vi "Search.vi"(8 "error in (no error)":errorcluster, 9 "SearchMethod":T1, 11 "MultiTree in":refnum<class "MultiTree.lvclass">) -> (0 "error out":errorcluster, 1 "found":bool, 2 "Node":refnum<data-value>, 3 "MultiTree out":refnum<class "MultiTree.lvclass">)   [LabVIEW 2014, in "MultiTree.lvlib" / "MultiTree.lvclass"]
uses:
  <userlib>/AdvancedDataStructures/ClassBased/MultiTree/MultiTree.lvclass
  <userlib>/AdvancedDataStructures/ClassBased/MultiTreeNode/MultiTreeNode.lvclass
  <userlib>/AdvancedDataStructures/ClassBased/MultiTree/SearchMethod.ctl
  <userlib>/AdvancedDataStructures/ClassBased/MultiTree/MultiTree.lvclass/MultiTree.ctl
  <userlib>/AdvancedDataStructures/ClassBased/MultiTreeNode/MultiTreeNode.lvclass/MultiTreeNode.ctl
  <userlib>/AdvancedDataStructures/ClassBased/LinkedList/LinkedList.lvclass
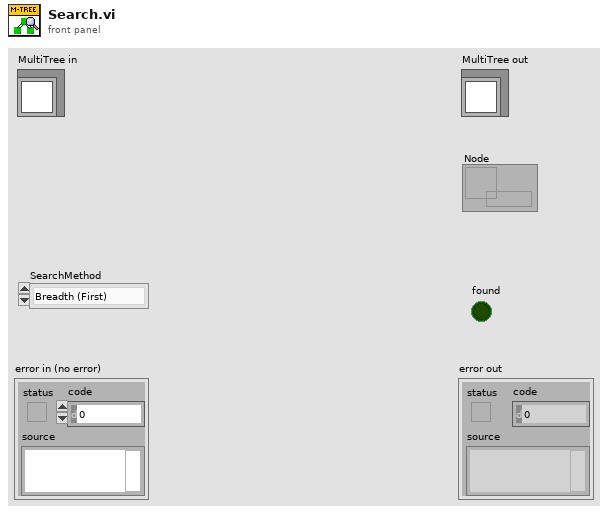
[diagram p1: front panel]
types:
  T1 = typedef "MultiTree.lvlib/MultiTree.lvclass/SearchMethod.ctl" = enum16{"Breadth (First)", "Depth (First)", "Best First", "Breadth (Exhaustive)", "Depth (Exhaustive)"}
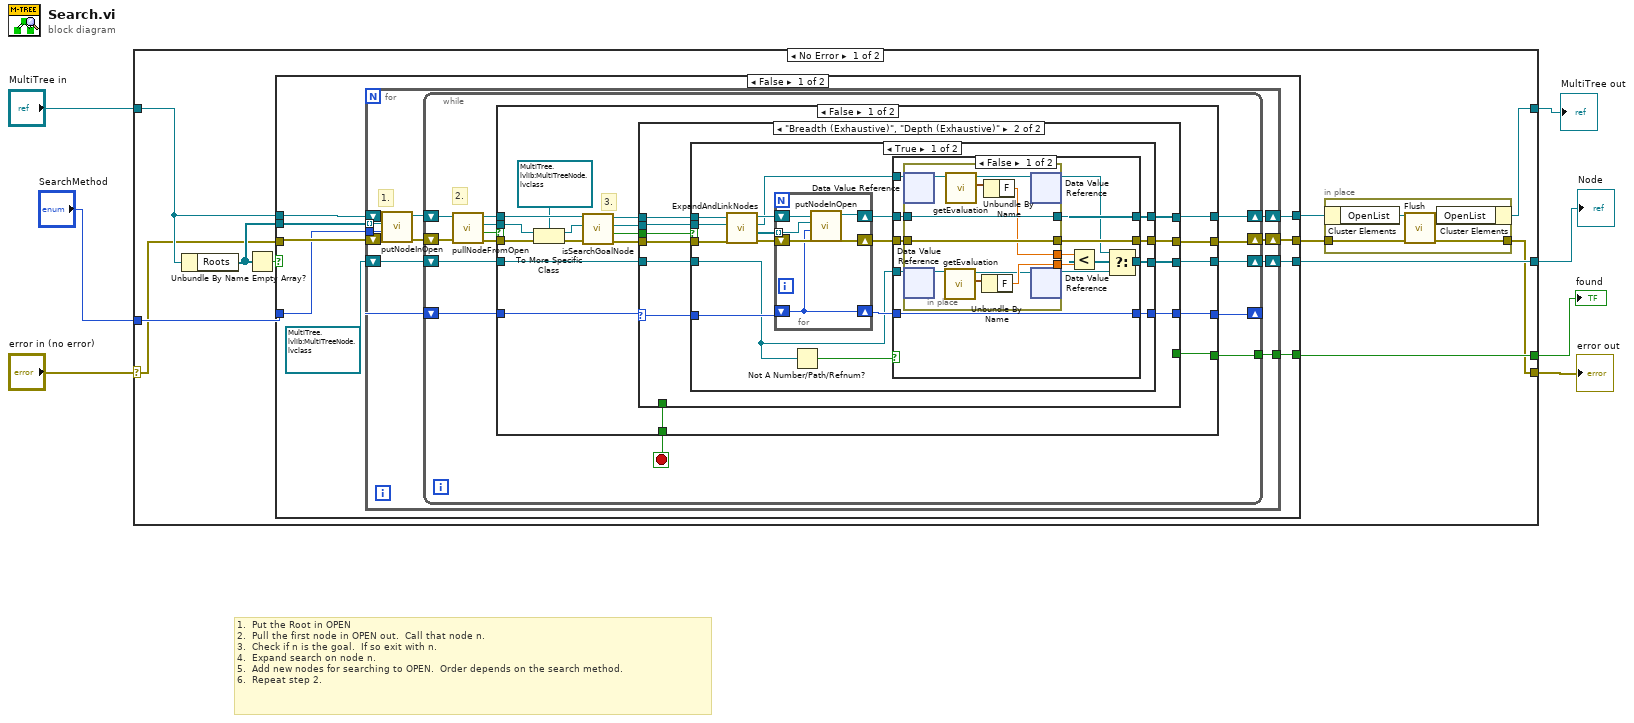
[diagram p0: block diagram]
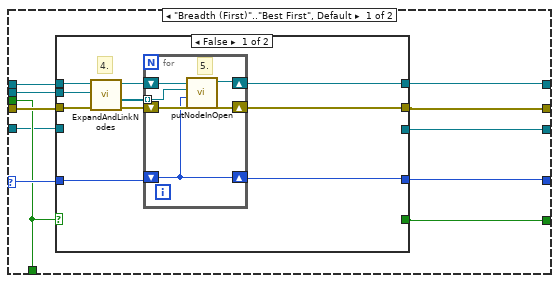
[diagram p2: hidden frame]
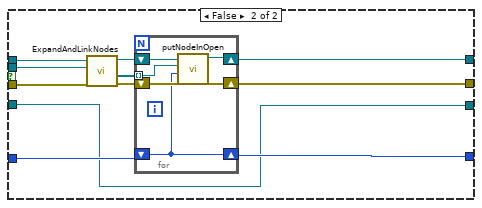
[diagram p5: hidden frame]
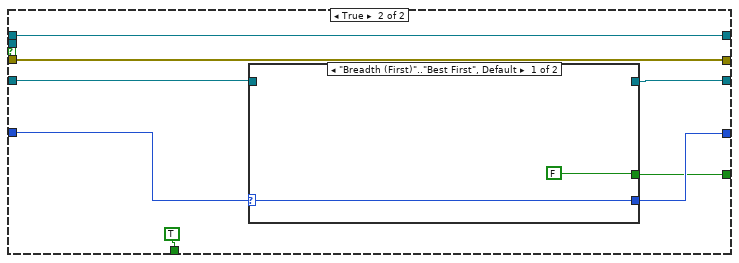
[diagram p6: hidden frame]
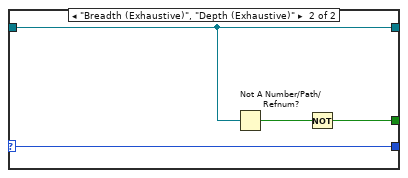
[diagram p7: hidden frame]
diagram:
  # "1.  Put the Root in OPEN\n2.  Pull the first node in OPEN out.  Call that node n.\n3.  Check if n is the goal.  If so exit with n.\n4.  Expand search on node n.\n5.  Add new nodes for searching to OPEN.  Order depends on the search method.\n6.  Repeat step 2."
  n1 = case shown="No Error" "error in (no error)" {
    selector: "error in (no error)" -> [w12 w201]
    tunnel: [w8 w201] -> w6
    tunnel: [w11 w200] -> w4
    tunnel: "MultiTree in" -> [w14 w200]
    tunnel: "SearchMethod" -> [w13 _]
    tunnel: [w10 _] -> w2
    tunnel: [w9 _] -> w1
    frame No Error {
      n2 = Unbundle By Name(w14) -> ("Roots"=w17:refnum<data-value>[])
      n3 = Empty Array?(array=w17) -> (empty?=w18:bool)
      n4 = case shown="False" w18 {
        tunnel: w14 -> [w31 w198]
        tunnel: w17 -> [w30 _]
        tunnel: w12 -> [w29 w199]
        tunnel: [w27 w198] -> w15
        tunnel: [w26 w199] -> w16
        tunnel: [w28 _] -> w9
        tunnel: w13 -> [w24 _]
        tunnel: [w25 _] -> w10
        frame False {
          n5 = for {
            tunnel: w30 -> [w40] mode=indexing
            tunnel: [w37] -> w28
            tunnel: w24 -> [w33]
            shift-right: [w36] -> w27
            shift-left: w31 -> [w42]
            shift-right: [w35] -> w26
            shift-left: w29 -> [w39]
            shift-right: [w34] -> w25
            shift-left: refnum<data-value> refnum ("NodeToIdentify out") -> [w32]
            # "1."
            n6 = call <userlib>:"putNodeInOpen.vi"("error in (no error)"=w39, "SearchMethod"=w33, "MultiTreeNode"=w40, "MultiTree in"=w42) -> ("error out"=w38:errorcluster, "MultiTree out"=w41:refnum<class "MultiTree.lvclass">)  [unwired: 6 in]
            n7 = while {
              shift-right: [w50] -> w36
              shift-left: w41 -> [w43]
              shift-right: [w49] -> w35
              shift-left: w38 -> [w56]
              tunnel: [w51] -> w37
              shift-right: [w46] -> _
              shift-left: w33 -> [w47]
              shift-right: [w48] -> w34
              shift-left: w32 -> [w44]
              stop <- w54 stop-if-true
              # "2."
              n8 = call <userlib>:"pullNodeFromOpen.vi"("error in (no error)"=w56, "MultiTree in"=w43) -> ("error out"=w55:errorcluster, "empty"=w53:bool, "RemovedNode"=w45:refnum<data-value>, "MultiTree out"=w52:refnum<class "MultiTree.lvclass">)  [unwired: 6 in]
              n9 = case shown="False" w53 {
                tunnel: w55 -> [w71 w189]
                tunnel: [w65 TRUE ("found")] -> w54
                tunnel: w52 -> [w74 w190]
                tunnel: [w57 w186] -> w51
                tunnel: [w59 w190] -> w50
                tunnel: [w60 w189] -> w49
                tunnel: [w58 w184] -> w48
                tunnel: w47 -> [w68 w188]
                tunnel: [w61 w187] -> w46
                tunnel: w45 -> [w72 _]
                tunnel: w44 -> [w67 w185]
                frame False {
                  # "3."
                  n10 = To More Specific Class(target class=refnum<data-value> refnum ("Node"), reference=w72, error in=w71) -> (specific class reference=w69:refnum<data-value>, error out=w70:errorcluster)
                  n11 = call-dynamic "isSearchGoalNode.vi"("error in (no error)"=w70, "PossibleSearchGoal in"=w69, "MultiTree in"=w74) -> ("error out"=w64:errorcluster, "IsNode"=w66:bool, "PossibleSearchGoal out"=w63:refnum<data-value>, "MultiTree out"=w62:refnum<class "MultiTree.lvclass">)  [unwired: 5 in]
                  n12 = case shown="\"Breadth (Exhaustive)\", \"Depth (Exhaustive)\"" w68 {
                    selector: w68 -> [w85 w115]
                    tunnel: [w80 w113] -> w61
                    tunnel: w67 -> [w76 w108]
                    tunnel: w66 -> [w77 w111]
                    tunnel: [w77 _] -> w65
                    tunnel: [w78 w107] -> w58
                    tunnel: w64 -> [w81 w112]
                    tunnel: w63 -> [w82 w114]
                    tunnel: w62 -> [w84 w116]
                    tunnel: [w83 w110] -> w59
                    tunnel: [w79 w109] -> w60
                    tunnel: [w75 _] -> w57
                    frame "Breadth (First)".."Best First", Default {
                      n13 = case shown="False" w77 {
                        selector: w77 -> [_ w106]
                        tunnel: [_ w106] -> w75
                        tunnel: w84 -> [w92 w105]
                        tunnel: [w94 w105] -> w83
                        tunnel: [w93 w103] -> w79
                        tunnel: w82 -> [w88 w102]
                        tunnel: w85 -> [w95 w104]
                        tunnel: [w87 w104] -> w80
                        tunnel: w81 -> [w86 w103]
                        tunnel: [_ w102] -> w78
                        tunnel: w76 -> [_ _]
                        frame False {
                          # "4."
                          n14 = call <userlib>:"ExpandAndLinkNodes.vi"("error in (no error)"=w86, "ToExpand in"=w88, "MultiTree in"=w92) -> ("error out"=w90:errorcluster, "ExpandedSearchNodes"=w89:refnum<data-value>[], "MultiTree out"=w91:refnum<class "MultiTree.lvclass">)  [unwired: 5 in, 1 out]
                          n15 = for {
                            shift-right: [w99] -> w94
                            shift-left: w91 -> [w101]
                            tunnel: w89 -> [w100] mode=indexing
                            shift-right: [w97] -> w93
                            shift-left: w90 -> [w98]
                            shift-right: [w96] -> w87
                            shift-left: w95 -> [w96]
                            # "5."
                            n16 = call <userlib>:"putNodeInOpen.vi"("error in (no error)"=w98, "SearchMethod"=w96, "MultiTreeNode"=w100, "MultiTree in"=w101) -> ("error out"=w97:errorcluster, "MultiTree out"=w99:refnum<class "MultiTree.lvclass">)  [unwired: 6 in]
                          }
                        }
                        frame True {
                        }
                      }
                    }
                    frame "Breadth (Exhaustive)", "Depth (Exhaustive)" {
                      n17 = case shown="True" w111 {
                        tunnel: w116 -> [w130 w174]
                        tunnel: w115 -> [w129 w173]
                        tunnel: w114 -> [w128 w172]
                        tunnel: [w118 w171] -> w113
                        tunnel: w112 -> [w127 w170]
                        tunnel: [w123 w169] -> w110
                        tunnel: [w122 w168] -> w109
                        tunnel: w108 -> [w117 w167]
                        tunnel: [w121 w167] -> w107
                        frame True {
                          n18 = call <userlib>:"ExpandAndLinkNodes.vi"("error in (no error)"=w127, "ToExpand in"=w128, "MultiTree in"=w130) -> ("error out"=w132:errorcluster, "ExpandedSearchNodes"=w131:refnum<data-value>[], "ToExpand out"=w126:refnum<data-value>, "MultiTree out"=w133:refnum<class "MultiTree.lvclass">)  [unwired: 5 in]
                          n19 = for {
                            shift-right: [w164] -> w124
                            shift-left: w133 -> [w166]
                            tunnel: w131 -> [w165] mode=indexing
                            shift-right: [w162] -> w125
                            shift-left: w132 -> [w163]
                            shift-right: [w161] -> w119
                            shift-left: w129 -> [w161]
                            n20 = call <userlib>:"putNodeInOpen.vi"("error in (no error)"=w163, "SearchMethod"=w161, "MultiTreeNode"=w165, "MultiTree in"=w166) -> ("error out"=w162:errorcluster, "MultiTree out"=w164:refnum<class "MultiTree.lvclass">)  [unwired: 6 in]
                          }
                          n21 = Not A Number/Path/Refnum?(number/path/refnum=w117) -> (NaN/Path/Refnum?=w120:bool)
                          n22 = case shown="False" w120 {
                            tunnel: w126 -> [w146 w157]
                            tunnel: w125 -> [w145 w159]
                            tunnel: w124 -> [w144 w160]
                            tunnel: [w143 w160] -> w123
                            tunnel: [w142 w159] -> w122
                            tunnel: [w136 w157] -> w121
                            tunnel: w119 -> [w135 w158]
                            tunnel: [w135 w158] -> w118
                            tunnel: w117 -> [w134 _]
                            frame False {
                              n23 = in-place {
                                in-place-border: w145 -> [w156]
                                in-place-border: [w156] -> w142
                                in-place-border: w144 -> [w155]
                                in-place-border: [w155] -> w143
                                in-place-border: [w150] -> w141
                                in-place-border: [w148] -> w140
                                n24 = in-place-dvr #1(w146) -> (w153:refnum<class "MultiTreeNode.lvclass">)  [unwired: 1 out]
                                n25 = in-place-dvr #2(w134) -> (w154:refnum<class "MultiTreeNode.lvclass">)  [unwired: 1 out]
                                n26 = call <userlib>:"getEvaluation.vi"("MultiTreeNode in"=w154) -> ("evaluation"=w149:cluster{"F":dbl, "G":dbl, "H":dbl}, "MultiTreeNode out"=w147:refnum<class "MultiTreeNode.lvclass">)  [unwired: 8 in, 1 out]
                                n27 = call <userlib>:"getEvaluation.vi"("MultiTreeNode in"=w153) -> ("evaluation"=w151:cluster{"F":dbl, "G":dbl, "H":dbl}, "MultiTreeNode out"=w152:refnum<class "MultiTreeNode.lvclass">)  [unwired: 8 in, 1 out]
                                n28 = Unbundle By Name(w149) -> ("F"=w148:dbl)
                                n29 = Unbundle By Name(w151) -> ("F"=w150:dbl)
                                n30 = in-place-dvr #1(w152) -> (w138:refnum<data-value>)  [unwired: 1 out]
                                n31 = in-place-dvr #2(w147) -> (w137:refnum<data-value>)  [unwired: 1 out]
                              }
                              n32 = Less?(x=w141, y=w140) -> (x < y?=w139:bool)
                              n33 = Select(t=w138, s=w139, f=w137) -> (s? t:f=w136:refnum<data-value>)
                            }
                            frame True {
                            }
                          }
                        }
                        frame False {
                          n34 = call <userlib>:"ExpandAndLinkNodes.vi"("error in (no error)"=w170, "ToExpand in"=w172, "MultiTree in"=w174) -> ("error out"=w176:errorcluster, "ExpandedSearchNodes"=w175:refnum<data-value>[], "MultiTree out"=w177:refnum<class "MultiTree.lvclass">)  [unwired: 5 in, 1 out]
                          n35 = for {
                            shift-right: [w181] -> w169
                            shift-left: w177 -> [w183]
                            tunnel: w175 -> [w182] mode=indexing
                            shift-right: [w179] -> w168
                            shift-left: w176 -> [w180]
                            shift-right: [w178] -> w171
                            shift-left: w173 -> [w178]
                            n36 = call <userlib>:"putNodeInOpen.vi"("error in (no error)"=w180, "SearchMethod"=w178, "MultiTreeNode"=w182, "MultiTree in"=w183) -> ("error out"=w179:errorcluster, "MultiTree out"=w181:refnum<class "MultiTree.lvclass">)  [unwired: 6 in]
                          }
                        }
                      }
                    }
                  }
                }
                frame True {
                  n37 = case shown="\"Breadth (First)\"..\"Best First\", Default" w188 {
                    selector: w188 -> [w193 w197]
                    tunnel: [w193 w197] -> w187
                    tunnel: [FALSE w194] -> w186
                    tunnel: w185 -> [_ w196]
                    tunnel: [_ w196] -> w184
                    frame "Breadth (First)".."Best First", Default {
                    }
                    frame "Breadth (Exhaustive)", "Depth (Exhaustive)" {
                      n38 = Not A Number/Path/Refnum?(number/path/refnum=w196) -> (NaN/Path/Refnum?=w195:bool)
                      n39 = Not(x=w195) -> (.not. x?=w194:bool)
                    }
                  }
                }
              }
            }
          }
        }
        frame True {
          # "No nodes in tree.  Cannot be found."
        }
      }
      n40 = in-place {
        in-place-border: w16 -> [w22]
        in-place-border: [w21] -> w8
        n41 = in-place-cluster #3(w15) -> ("OpenList"=w20:refnum<class "BasicSortedList.lvclass">)
        n42 = call <userlib>:"Flush.vi"("error in (no error)"=w22, "LinkedList in"=w20) -> ("error out"=w21:errorcluster, "LinkedList out"=w19:refnum<class "BasicSortedList.lvclass">)  [unwired: 7 in, 1 out]
        n43 = in-place-cluster #3("OpenList"=w19) -> (w11:refnum<class "MultiTree.lvclass">)
      }
    }
    frame Error {
    }
  }
  "error out" <- w6
  "MultiTree out" <- w4
  "Node" <- w2
  "found" <- w1
